vi "State_Queue_Driver.vi"(0 "Queue_Name_In":string, 1 "Max_Queue_Size_In":i32=-1, 5 "State_In":string, 7 "N_State_In":string[](array[string]), 9 "Time_Out_In_ms (10)":i32=10, 11 "Error_In":errorcluster, 13 "Queue_Operation":T1=enum."Flush") -> (3 "Max_Queue_Size_Out":i32=-1, 4 "Queue_Name_Out":string, 6 "State_Out":string, 15 "Error_Out":errorcluster)   [LabVIEW 2023]
doc: "Used to transfer data from one vi to another using queue."
uses:
  Controls/Queue_Driver_Select.ctl
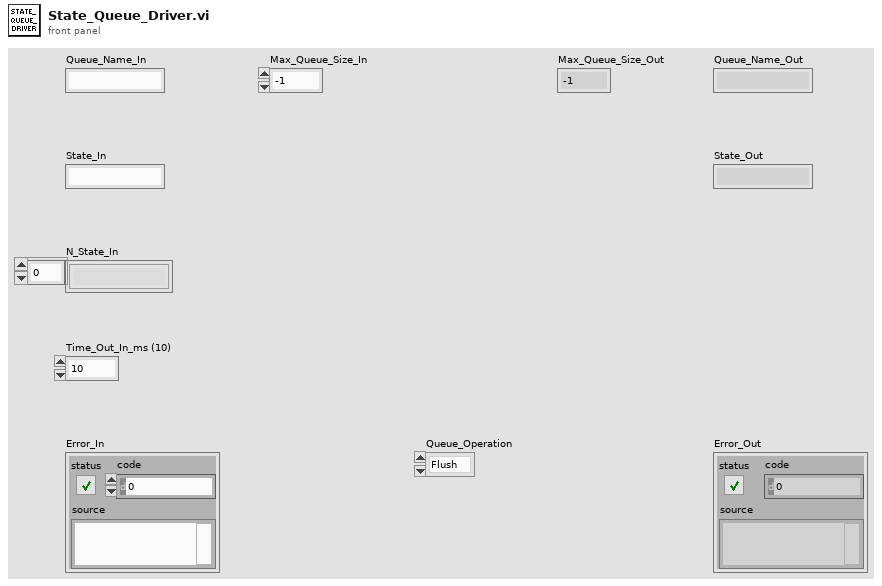
[diagram p1: front panel]
types:
  T1 = typedef "Queue_Driver_Select.ctl" = enum16{"Obtain_Queue", "Enqueue", "Enqueue_N", "Enqueue_at_End", "Preview", "Queue_Status", "Dequeue", "Flush", "Release_Queue"}
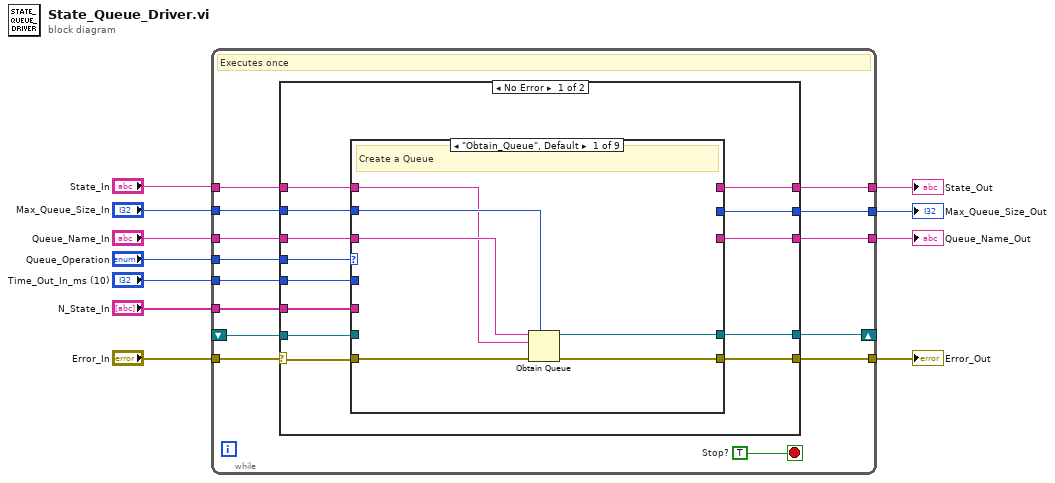
[diagram p0: block diagram]
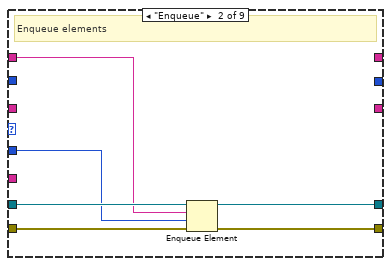
[diagram p2: hidden frame]
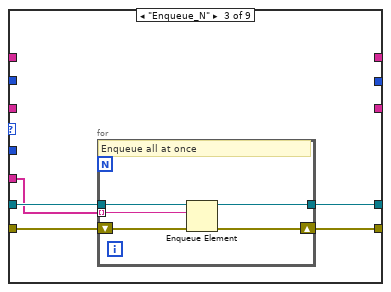
[diagram p3: hidden frame]
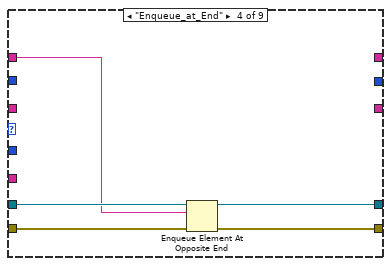
[diagram p4: hidden frame]
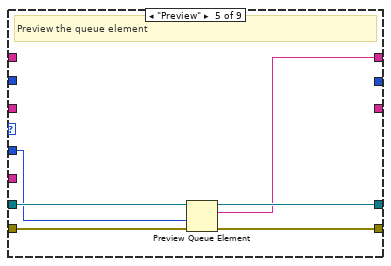
[diagram p5: hidden frame]
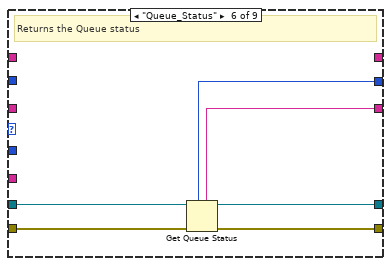
[diagram p6: hidden frame]
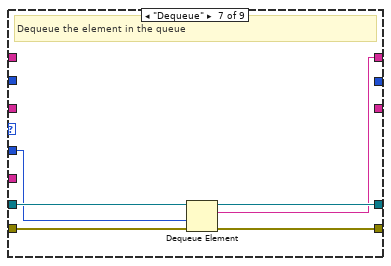
[diagram p7: hidden frame]
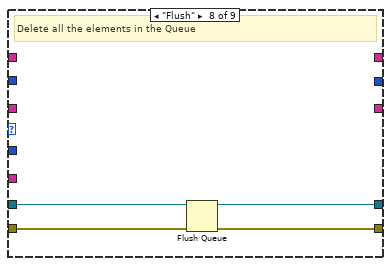
[diagram p8: hidden frame]
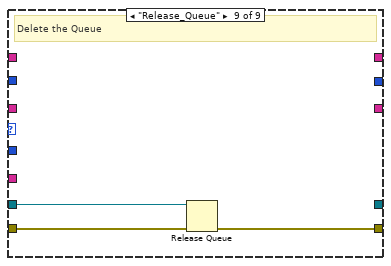
[diagram p9: hidden frame]
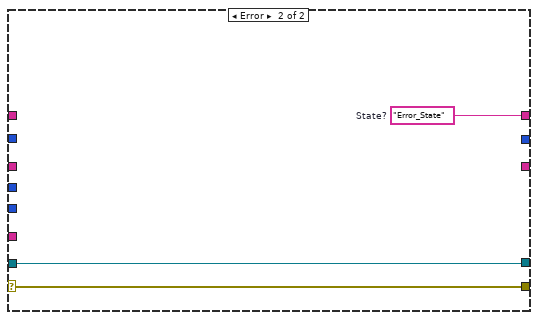
[diagram p10: hidden frame]
diagram:
  n1 = while {
    tunnel: "Max_Queue_Size_In" -> [w25]
    tunnel: "Time_Out_In_ms (10)" -> [w22]
    tunnel: [w20] -> w8
    tunnel: "Queue_Operation" -> [w17]
    shift-right: [w18] -> _
    shift-left: _ -> [w14]
    tunnel: "Error_In" -> [w15]
    tunnel: [w24] -> w10
    tunnel: "N_State_In" -> [w12]
    tunnel: "State_In" -> [w23]
    tunnel: [w21] -> w2
    tunnel: "Queue_Name_In" -> [w16]
    tunnel: [w19] -> w7
    stop <- w13 stop-if-true
    w13 = TRUE  # Stop?
    # "Executes once"
    n2 = case shown="No Error" w15 {
      selector: w15 -> [w28 w93]
      tunnel: w17 -> [w29 _]
      tunnel: w16 -> [w30 _]
      tunnel: w25 -> [w38 _]
      tunnel: [w37 w91] -> w18
      tunnel: [w36 w93] -> w24
      tunnel: w23 -> [w31 _]
      tunnel: w22 -> [w35 _]
      tunnel: [w34 w92] -> w21
      tunnel: [w33 _] -> w20
      tunnel: [w32 _] -> w19
      tunnel: w14 -> [w27 w91]
      tunnel: w12 -> [w26 _]
      frame No Error {
        n3 = case shown="\"Obtain_Queue\", Default" w29 {
          tunnel: w28 -> [w44 w50 w51 w64 w70 w76 w82 w86 w89]
          tunnel: w30 -> [w42 _ _ _ _ _ _ _ _]
          tunnel: w38 -> [w41 _ _ _ _ _ _ _ _]
          tunnel: [w39 w46 w54 w63 w69 w75 w81 w85 _] -> w37
          tunnel: [w43 w49 w53 w62 w68 w74 w79 w84 w88] -> w36
          tunnel: w27 -> [_ w48 w55 w65 w71 w77 w83 w87 w90]
          tunnel: w31 -> [w40 w47 _ w61 _ _ _ _ _]
          tunnel: w35 -> [_ w45 _ _ w67 _ w78 _ _]
          tunnel: [_ _ _ _ w66 _ w80 _ _] -> w34
          tunnel: [_ _ _ _ _ w73 _ _ _] -> w33
          tunnel: [_ _ _ _ _ w72 _ _ _] -> w32
          tunnel: w26 -> [_ _ w52 _ _ _ _ _ _]
          frame "Obtain_Queue", Default {
            # "Create a Queue"
            n4 = Obtain Queue(max queue size (-1, unlimited)=w41, name (unnamed)=w42, element data type=w40, error in (no error)=w44) -> (queue out=w39:refnum<queue>, error out=w43:errorcluster)  [unwired: 1 in, 1 out]
          }
          frame "Enqueue" {
            # "Enqueue elements"
            n5 = Enqueue Element(queue=w48, element=w47, timeout in ms (-1)=w45, error in (no error)=w50) -> (queue out=w46:refnum<queue>, error out=w49:errorcluster)  [unwired: 1 out]
          }
          frame "Enqueue_N" {
            n6 = for {
              tunnel: w55 -> [w60]
              tunnel: [w58] -> w54
              shift-right: [w57] -> w53
              shift-left: w51 -> [w59]
              tunnel: w52 -> [w56] mode=indexing
              # "Enqueue all at once"
              n7 = Enqueue Element(queue=w60, element=w56, error in (no error)=w59) -> (queue out=w58:refnum<queue>, error out=w57:errorcluster)  [unwired: 1 in, 1 out]
            }
          }
          frame "Enqueue_at_End" {
            n8 = Enqueue Element At Opposite End(queue=w65, element=w61, error in (no error)=w64) -> (queue out=w63:refnum<queue>, error out=w62:errorcluster)  [unwired: 1 in, 1 out]
          }
          frame "Preview" {
            # "Preview the queue element"
            n9 = Preview Queue Element(queue=w71, timeout in ms (-1)=w67, error in (no error)=w70) -> (queue out=w69:refnum<queue>, element=w66:string, error out=w68:errorcluster)  [unwired: 1 out]
          }
          frame "Queue_Status" {
            # "Returns the Queue status"
            n10 = Get Queue Status(queue=w77, error in (no error)=w76) -> (queue out=w75:refnum<queue>, queue name=w72:string, max queue size=w73:i32, error out=w74:errorcluster)  [unwired: 1 in, 4 out]
          }
          frame "Dequeue" {
            # "Dequeue the element in the queue"
            n11 = Dequeue Element(queue=w83, timeout in ms (-1)=w78, error in (no error)=w82) -> (queue out=w81:refnum<queue>, element=w80:string, error out=w79:errorcluster)  [unwired: 1 out]
          }
          frame "Flush" {
            # "Delete all the elements in the Queue"
            n12 = Flush Queue(queue=w87, error in (no error)=w86) -> (queue out=w85:refnum<queue>, error out=w84:errorcluster)  [unwired: 1 out]
          }
          frame "Release_Queue" {
            # "Delete the Queue"
            n13 = Release Queue(queue=w90, error in (no error)=w89) -> (error out=w88:errorcluster)  [unwired: 1 in, 2 out]
          }
        }
      }
      frame Error {
        w92 = "Error_State"  # State?
      }
    }
  }
  "Error_Out" <- w10
  "Max_Queue_Size_Out" <- w8
  "Queue_Name_Out" <- w7
  "State_Out" <- w2
